vi "NetComm_CAN_ReadStreamSession.vi"(8 "error in (no error)":errorcluster, 10 "Messages To Read":u32, 11 "Session Handle":u32) -> (0 "error out":errorcluster, 2 "Messages":T1(array[cluster]) {"Message ID" format="%.0x"; "Data" format="%.0x"}, 3 "Session Handle Out":u32)   [LabVIEW 2017]
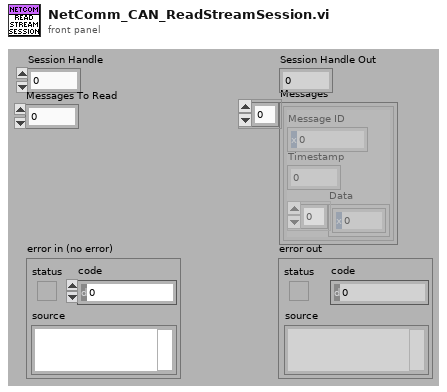
[diagram p1: front panel]
types:
  T1 = cluster{"Message ID":u32, "Timestamp":u32, "Data":u8[]}[]
  T2 = enum16{"big-endian, network order", "native, host order", "little-endian"}
  T3 = cluster{"Message ID":u32, "Timestamp":u32, "Data":u8[]}
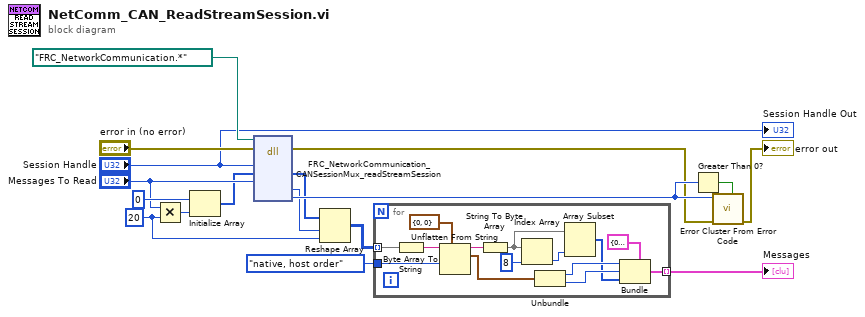
[diagram p0: block diagram]
diagram:
  w4 = u32 20 ("x")
  n1 = Multiply(x="Messages To Read", y=w4) -> (x*y=w8:u32)
  n2 = Initialize Array(u8 0, w8) -> (w7:u8[])
  n3 = dll-call lib="FRC_NetworkCommunication.*" fn="FRC_NetworkCommunication_CANSessionMux_readStreamSession"(path in=path "FRC_NetworkCommunication.*", error in="error in (no error)", "sessionHandle"="Session Handle", "messages"=w7, "messagesToRead"="Messages To Read") -> (error out=w13:errorcluster, "messages"=w6:u8[], "messagesRead"=w5:u32, "status"=w14:i32)  [unwired: 6 in, 1 out]
  n4 = Reshape Array(w6, w5, w4) -> (w3:u8[][])
  n5 = for {
    tunnel: w3 -> [w31] mode=indexing
    tunnel: T2."native, host order" ("byte order (0:big-endian, network order)") -> [w28]
    tunnel: [w18] -> w1 mode=indexing
    n6 = Byte Array To String(unsigned byte array=w31) -> (string=w30:string)
    n7 = Unflatten From String(type=cluster{"Message ID":u32, "Timestamp":u32} {"Message ID"=0, "Timestamp"=0}, binary string=w30, byte order (0:big-endian, network order)=w28) -> (rest of the binary string=w27:string, value=w23:cluster{"Message ID":u32, "Timestamp":u32})  [unwired: 2 in, 1 out]
    n8 = String To Byte Array(string=w27) -> (unsigned byte array=w24:u8[])
    n9 = Index Array(array=w24, index=8) -> (element=w25:u8)
    n10 = Unbundle(w23) -> ("Message ID"=w21:u32, "Timestamp"=w20:u32)
    n11 = Array Subset(array=w24, length=w25) -> (w19:u8[])  [unwired: 1 in]
    n12 = Bundle(cluster=T3 {"Message ID"=0, "Timestamp"=0, "Data"=[]}, "Message ID"=w21, "Timestamp"=w20, "Data"=w19) -> (w18:T3)
  }
  "Messages" <- w1
  n13 = Greater Than 0?(x=w14) -> (x > 0?=w15:bool)
  n14 = call <vilib>:"Error Cluster From Error Code.vi"("is warning? (False)"=w15, "error in (no error)"=w13, "error code (0)"=w14) -> ("error out"=→"error out":errorcluster)  [unwired: 1 in, 5 out]
  "Session Handle Out" <- "Session Handle"
